vi "Amium String zerlegen.vi"(5 "read buffer":string) -> (6 "Array":string[](array[string]))   [LabVIEW 2020, in "Amium PNS.lvlib" / "AK Kommunikation.lvlib"]
uses:
  AK Kommunikation.lvlib
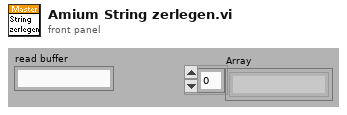
[diagram p1: front panel]
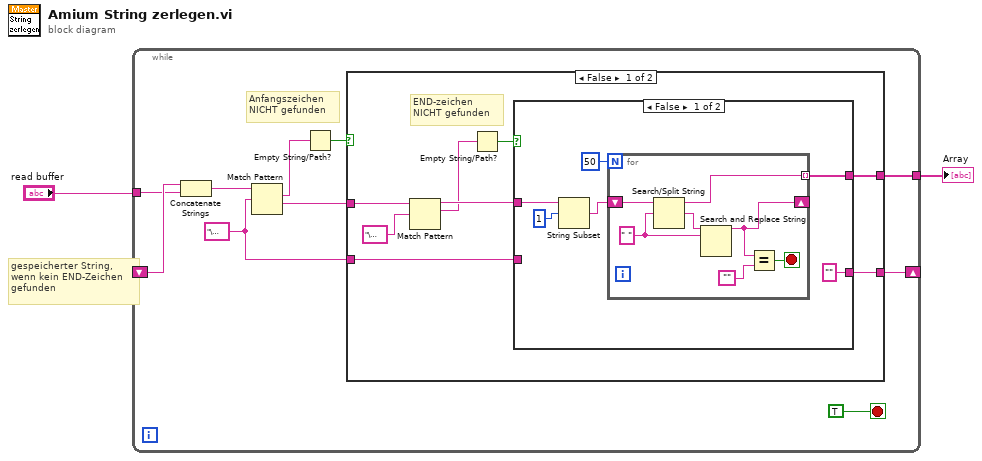
[diagram p0: block diagram]
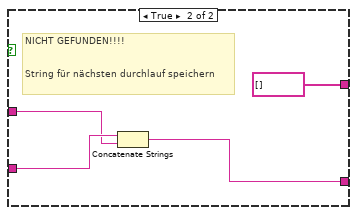
[diagram p2: hidden frame]
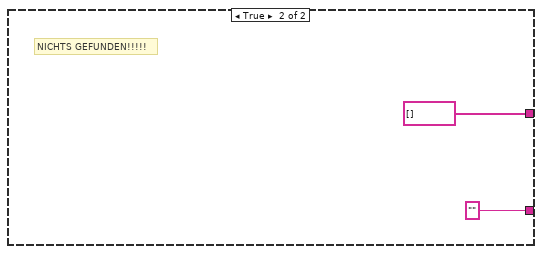
[diagram p3: hidden frame]
diagram:
  # "gespeicherter String,\nwenn kein END-Zeichen\ngefunden"
  n1 = while {
    shift-right: [w9] -> _
    shift-left: _ -> [w8]
    tunnel: "read buffer" -> [w7]
    tunnel: [w5] -> w1
    stop <- TRUE stop-if-true
    w11 = "\u0002" ("String")
    # "Anfangszeichen \nNICHT gefunden"
    n2 = Concatenate Strings(w8, w7) -> (w6:string)
    n3 = Match Pattern(string=w6, regular expression=w11) -> (match substring=w3:string, after substring=w12:string)  [unwired: 1 in, 2 out]
    n4 = Empty String/Path?(string/path=w3) -> (empty?=w4:bool)
    n5 = case shown="False" w4 {
      tunnel: [w20 string[] []] -> w5
      tunnel: w12 -> [w19 _]
      tunnel: w11 -> [w16 _]
      tunnel: [w15 ""] -> w9
      frame False {
        # "END-zeichen \nNICHT gefunden"
        n6 = Match Pattern(string=w19, regular expression="\u0003" ("String")) -> (before substring=w17:string, match substring=w14:string)  [unwired: 1 in, 2 out]
        n7 = Empty String/Path?(string/path=w14) -> (empty?=w13:bool)
        n8 = case shown="False" w13 {
          tunnel: [w26 string[] []] -> w20
          tunnel: w17 -> [w22 w36]
          tunnel: w16 -> [_ w37]
          tunnel: ["" w35] -> w15
          frame False {
            n9 = String Subset(string=w22, offset (0)=1 ("Offset (0)")) -> (substring=w21:string)  [unwired: 1 in]
            n10 = for {
              N: 50 -> [_]
              shift-right: [w28] -> _
              shift-left: w21 -> [w33]
              tunnel: [w32] -> w26 mode=indexing
              stop <- w27 stop-if-true
              w30 = " " ("Nach String/Zeichen suchen (-)")
              n11 = Search/Split String(string=w33, search string/char (-)=w30) -> (substring before match=w32:string, match + rest of string=w31:string)  [unwired: 1 in, 1 out]
              n12 = Search and Replace String(input string=w31, search string=w30) -> (result string=w28:string)  [unwired: 6 in, 3 out]
              n13 = Equal?(x=w28, y="") -> (x = y?=w27:bool)
            }
          }
          frame True {
            # "NICHT GEFUNDEN!!!!\n\n\nString für nächsten durchlauf speichern"
            n14 = Concatenate Strings(w37, w36) -> (w35:string)
          }
        }
      }
      frame True {
        # "NICHTS GEFUNDEN!!!!!"
      }
    }
  }
  "Array" <- w1
